vi "Control Test.vi"() -> ()   [LabVIEW 2015, in "Peltier.lvclass"]
uses:
  Peltier.lvclass
  Typedefs/Peltier Temperature Sensors.ctl
panel:
  out "Set Point":dbl
  out "Kd":u8
  out "Ki":u8
  out "Kp":u8
  out "After":dbl[](array[numeric])
  out "Before":dbl[](array[numeric])
  in  "stop":bool
  out "error out":errorcluster
  out "Ready?":bool
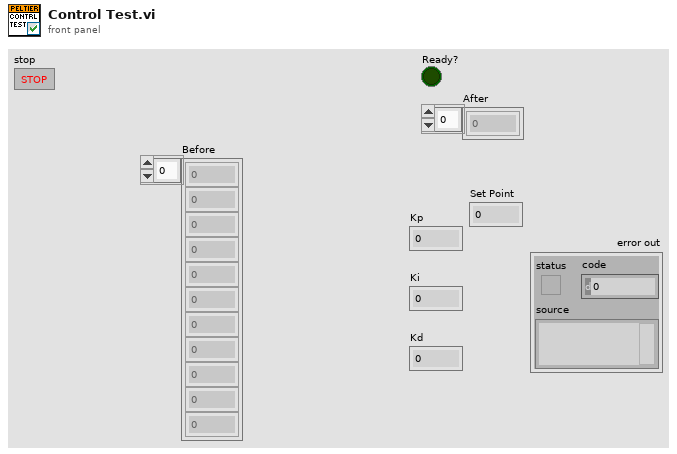
[diagram p1: front panel]
types:
  T1 = typedef "Peltier.lvclass/Peltier Temperature Sensors.ctl" = u16
  T2 = typedef "Peltier.lvclass/Session Handle.ctl" = refnum<data-value>
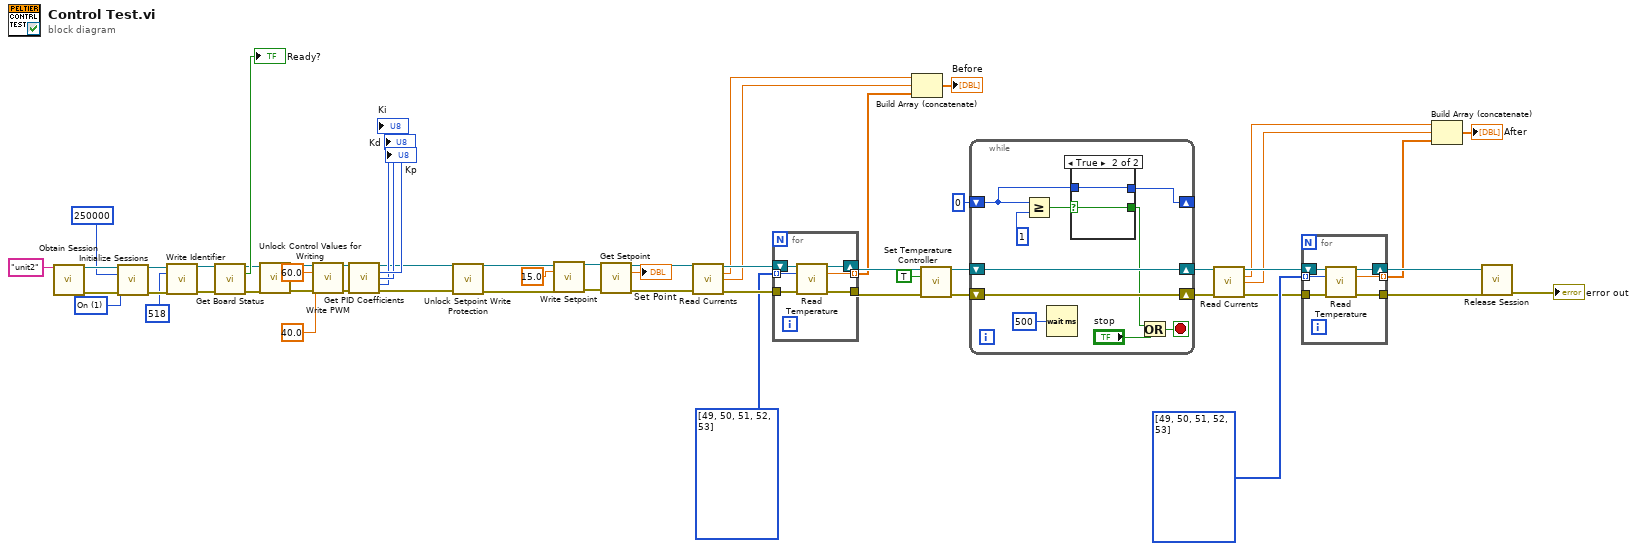
[diagram p0: block diagram]
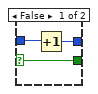
[diagram p2: hidden frame]
diagram:
  w39 = T1[] [49, 50, 51, 52, 53] items=["PTS1"=49, "PTS2"=50, "PTS3"=51, "PTS4"=52, "PTS5"=53, "PTS6"=54]
  w43 = T1[] [49, 50, 51, 52, 53] items=["PTS1"=49, "PTS2"=50, "PTS3"=51, "PTS4"=52, "PTS5"=53, "PTS6"=54]
  w53 = u32 1 items=["Off", "On"] ("Termination")
  n1 = call "Obtain Session.vi"("Session  Name ()"="unit2") -> ("Session Handle"=w56:T2, "error out"=w55:errorcluster)  [unwired: 13 in]
  n2 = call "Initialize Sessions.vi"("Session Handle"=w56, "Baud Rate"=u32 250000, "Termination"=w53, "error in (no error)"=w55) -> ("Session Handle Out"=w52:T2, "error out"=w51:errorcluster)  [unwired: 10 in]
  n3 = call "Write Identifier.vi"("Session Handle In"=w52, "identifier"=u16 518, "error in (no error)"=w51) -> ("Session Handle Out"=w49:T2, "error out"=w48:errorcluster)  [unwired: 11 in]
  n4 = call "Get Board Status.vi"("Session Handle"=w49, "error in (no error)"=w48) -> ("Session Handle Out"=w26:T2, "Ready?"=→"Ready?":bool, "error out"=w25:errorcluster)  [unwired: 11 in]
  n5 = call "Unlock Control Values for Writing.vi"("Session Handle"=w26, "error in (no error)"=w25) -> ("Session Handle Out"=w24:T2, "error out"=w23:errorcluster)  [unwired: 12 in]
  n6 = call "Write PWM.vi"("Session Handle"=w24, "Max PWM"=60.0, "Min PWM"=40.0, "error in (no error)"=w23) -> ("Session Handle Out"=w15:T2, "error out"=w14:errorcluster)  [unwired: 10 in]
  n7 = call "Get PID Coefficients.vi"("Session Handle"=w15, "error in (no error)"=w14) -> ("Session Handle Out"=w4:T2, "Kp"=→"Kp":u8, "Ki"=→"Ki":u8, "Kd"=→"Kd":u8, "error out"=w2:errorcluster)  [unwired: 9 in]
  n8 = call "Unlock Setpoint Write Protection.vi"("Session Handle"=w4, "error in (no error)"=w2) -> ("Session Handle Out"=w3:T2, "error out"=w1:errorcluster)  [unwired: 12 in]
  n9 = call "Write Setpoint.vi"("Session Handle"=w3, "Setpoint"=15.0, "error in (no error)"=w1) -> ("Session Handle Out"=w6:T2, "error out"=w5:errorcluster)  [unwired: 11 in]
  n10 = call "Get Setpoint.vi"("Session Handle"=w6, "error in (no error)"=w5) -> ("Session Handle Out"=w9:T2, "Set Point"=→"Set Point":dbl, "error out"=w10:errorcluster)  [unwired: 11 in]
  n11 = call "Read Currents.vi"("Session Handle"=w9, "error in (no error)"=w10) -> ("Session Handle Out"=w45:T2, "Side 1 Current"=w34:dbl, "Side 2 Current"=w33:dbl, "error out"=w44:errorcluster)  [unwired: 10 in]
  n12 = for {
    tunnel: w44 -> [w62]
    shift-right: [w59] -> w41
    shift-left: w45 -> [w63]
    tunnel: [w61] -> w42
    tunnel: w43 -> [w60] mode=indexing
    tunnel: [w58] -> w32 mode=indexing
    n13 = call "Read Temperature.vi"("Session Handle"=w63, "Pelt Temp Sensors"=w60, "error in (no error)"=w62) -> ("Session Handle Out"=w59:T2, "Temperature"=w58:dbl, "error out"=w61:errorcluster)  [unwired: 10 in]
  }
  n14 = Build Array (concatenate)(w34, w33, w32) -> (→"Before":dbl[])
  n15 = call "Set Temperature Controller.vi"("Session Handle"=w41, "On?"=TRUE, "error in (no error)"=w42) -> ("Session Handle Out"=w31:T2, "error out"=w30:errorcluster)  [unwired: 11 in]
  n16 = while {
    shift-right: [w73] -> w28
    shift-left: w31 -> [w73]
    shift-right: [w72] -> w27
    shift-left: w30 -> [w72]
    shift-right: [w65] -> _
    shift-left: 0 -> [w66]
    stop <- w64 stop-if-true
    n17 = Greater Or Equal?(x=w66, y=1) -> (x >= y?=w69:bool)
    n18 = Wait (ms)(milliseconds to wait=u32 500) -> ()  [unwired: 1 out]
    n19 = case shown="True" w69 {
      selector: w69 -> [w74 w78]
      tunnel: [w74 w78] -> w67
      tunnel: w66 -> [w76 w77]
      tunnel: [w75 w77] -> w65
      frame False {
        n20 = Increment(x=w76) -> (x+1=w75:i32)
      }
      frame True {
      }
    }
    n21 = Or(x=w67, y="stop") -> (x .or. y?=w64:bool)
  }
  n22 = call "Read Currents.vi"("Session Handle"=w28, "error in (no error)"=w27) -> ("Session Handle Out"=w37:T2, "Side 1 Current"=w19:dbl, "Side 2 Current"=w18:dbl, "error out"=w38:errorcluster)  [unwired: 10 in]
  n23 = for {
    tunnel: w38 -> [w83]
    shift-right: [w80] -> w35
    shift-left: w37 -> [w84]
    tunnel: [w82] -> w36
    tunnel: w39 -> [w81] mode=indexing
    tunnel: [w79] -> w17 mode=indexing
    n24 = call "Read Temperature.vi"("Session Handle"=w84, "Pelt Temp Sensors"=w81, "error in (no error)"=w83) -> ("Session Handle Out"=w80:T2, "Temperature"=w79:dbl, "error out"=w82:errorcluster)  [unwired: 10 in]
  }
  n25 = Build Array (concatenate)(w19, w18, w17) -> (→"After":dbl[])
  n26 = call "Release Session.vi"("Session Handle"=w35, "error in (no error)"=w36) -> ("error out"=→"error out":errorcluster)  [unwired: 13 in]
